vi "Read Configuration File.vi"(8 "error in (no error)":errorcluster, 11 "RP100 in":refnum<class "RP100.lvclass">) -> (0 "error out":errorcluster, 3 "RP100 out":refnum<class "RP100.lvclass">)   [LabVIEW 2019, in "RP100.lvclass"]
uses:
  RP100.lvclass
  <userlib>/LevyLab/Instrument Framework/SMOs/Instrument/Instrument.lvclass
  <userlib>/LevyLab/Instrument Framework/SMOs/Configuration/Configuration.lvclass
  C:/Program Files (x86)/National Instruments/LabVIEW 2019/user.lib/LevyLab/Instrument Framework/Instrument Types/Strain/Instrument.Strain.lvclass
  C:/Program Files (x86)/National Instruments/LabVIEW 2019/user.lib/LevyLab/Instrument Framework/SMOs/Instrument/Instrument.lvclass
  C:/Program Files (x86)/National Instruments/LabVIEW 2019/vi.lib/JKI/JKI SMO/SMO/SMO.lvclass
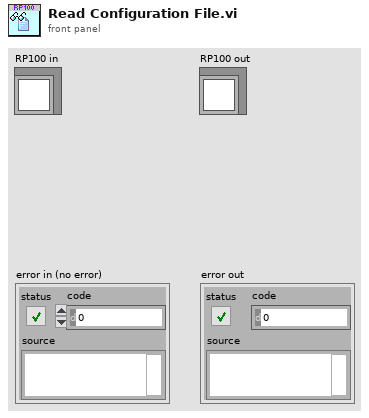
[diagram p1: front panel]
types:
  T1 = cluster{"RP100 Address":string, "C Bridge Address":string}
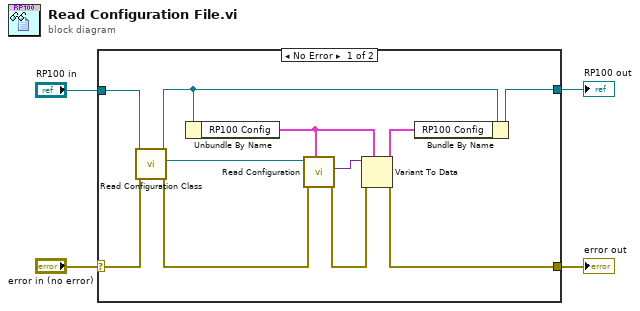
[diagram p0: block diagram]
diagram:
  n1 = case shown="No Error" "error in (no error)" {
    selector: "error in (no error)" -> [w12 w17]
    tunnel: [w11 w17] -> w1
    tunnel: [w15 w16] -> w3
    tunnel: "RP100 in" -> [w14 w16]
    frame No Error {
      n2 = call <userlib>:"Read Configuration Class.vi"("error in (no error)"=w12, "Instrument in"=w14) -> ("error out"=w9:errorcluster, "Configuration"=w8:refnum<class "Configuration.lvclass">, "Instrument out"=w13:refnum<class "RP100.lvclass">)  [unwired: 7 in]
      n3 = Unbundle By Name(w13) -> ("RP100 Config"=w10:T1)
      n4 = call <userlib>:"Read Configuration.vi"("INI Fomatted Cluster Type"=w10, "error in (no error)"=w9, "Configuration in"=w8) -> ("error out"=w6:errorcluster, "Configuration"=w7:variant)  [unwired: 6 in, 1 out]
      n5 = Variant To Data(error in=w6, type=w10, Variant=w7) -> (data=w5:T1, error out=w11:errorcluster)
      n6 = Bundle By Name(cluster=w13, "RP100 Config"=w5) -> (w15:refnum<class "RP100.lvclass">)
    }
    frame Error {
    }
  }
  "RP100 out" <- w3
  "error out" <- w1
